vi "String to Separate Chars.vi"(11 "String":string) -> (3 "Array":string[](array[string]))   [LabVIEW 2021]
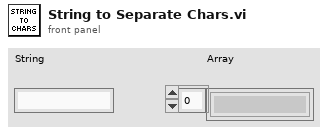
[diagram p1: front panel]
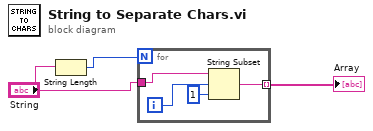
[diagram p0: block diagram]
diagram:
  n1 = String Length(string="String") -> (length=w1:i32)
  n2 = for {
    N: w1 -> [_]
    tunnel: "String" -> [w5]
    tunnel: [w4] -> w3 mode=indexing
    i -> [w7]
    n3 = String Subset(string=w5, offset (0)=w7, length (rest)=1 ("length (rest)")) -> (substring=w4:string)
  }
  "Array" <- w3
